vi "ROIsToPoints.vi"(9 "GridPoints":dbl=5.0, 10 "Scan Settings":T2, 11 "ROI":T1(array[cluster])) -> (0 "X-Y Motion Points":i32[][](array[numeric]), 1 "Number of motion points":i32, 2 "Number of points":i32, 3 "Points":i32[][](array[numeric]), 4 "Y-Z Motion Points":i32[][](array[numeric]))   [LabVIEW 2014]
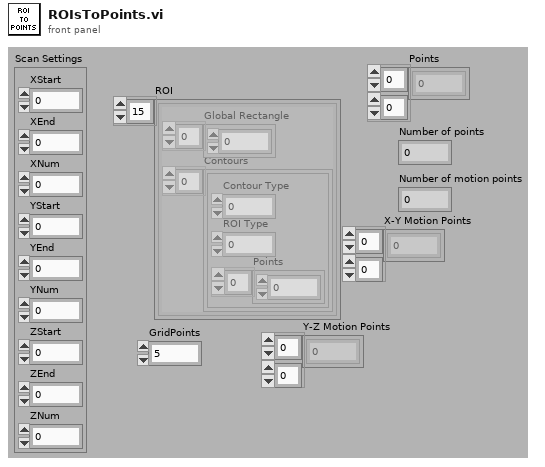
[diagram p1: front panel]
types:
  T1 = cluster{"Global Rectangle":i32[], "Contours":cluster{"Contour Type":u32, "ROI Type":u32, "Points":i32[]}[]}[]
  T2 = cluster{"XStart":i32, "XEnd":i32, "XNum":i32, "YStart":i32, "YEnd":i32, "YNum":i32, "ZStart":i32, "ZEnd":i32, "ZNum":i32}
  T3 = cluster{"Contour Type":u32, "ROI Type":u32, "Points":i32[]}[]
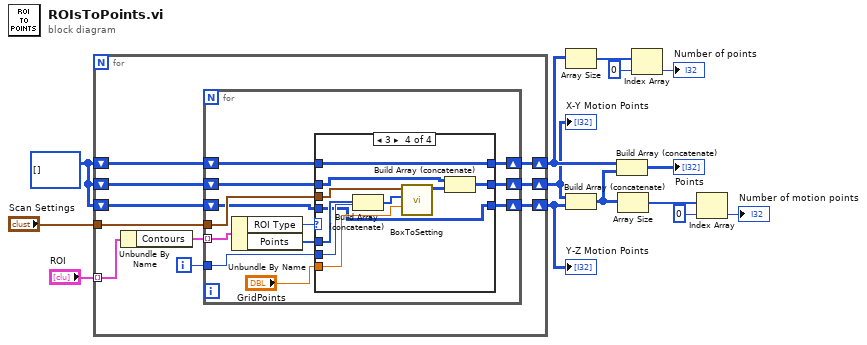
[diagram p0: block diagram]
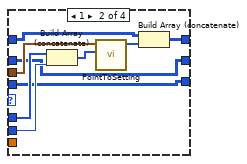
[diagram p3: hidden frame]
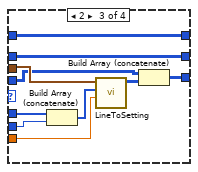
[diagram p4: hidden frame]
diagram:
  w4 = i32[][] []
  n1 = for {
    tunnel: "ROI" -> [w24] mode=indexing
    shift-right: [w20] -> w9
    shift-left: w4 -> [w21]
    tunnel: "Scan Settings" -> [w19]
    shift-right: [w15] -> w3
    shift-left: w4 -> [w18]
    shift-right: [w16] -> w2
    shift-left: w4 -> [w17]
    i -> [w22]
    n2 = Unbundle By Name(w24) -> ("Contours"=w23:T3)
    n3 = for {
      tunnel: w23 -> [w36] mode=indexing
      tunnel: w22 -> [w32]
      shift-right: [w31] -> w20
      shift-left: w21 -> [w33]
      tunnel: w19 -> [w30]
      shift-right: [w25] -> w15
      shift-left: w18 -> [w26]
      shift-right: [w27] -> w16
      shift-left: w17 -> [w28]
      n4 = Unbundle By Name(w36) -> ("ROI Type"=w35:u32, "Points"=w34:i32[])
      n5 = case shown="3" w35 {
        tunnel: w34 -> [_ w48 w58 w67]
        tunnel: w33 -> [w39 w46 w50 w59]
        tunnel: w32 -> [_ w47 w57 w68]
        tunnel: [w39 w45 w50 w59] -> w31
        tunnel: w30 -> [_ w43 w56 w66]
        tunnel: "GridPoints" -> [_ _ w54 w64]
        tunnel: w28 -> [w38 w41 w52 w62]
        tunnel: [w38 w41 w51 w62] -> w27
        tunnel: w26 -> [w37 w40 w49 w61]
        tunnel: [w37 w40 w49 w60] -> w25
        frame 0, Default {
        }
        frame 1 {
          n6 = Build Array (concatenate)(w48, w47) -> (w42:i32[])
          n7 = call "PointToSetting.vi"("Clicked"=w42, "Scan Settings"=w43) -> ("Setting"=w44:i32[])  [unwired: 9 in]
          n8 = Build Array (concatenate)(w46, w44) -> (w45:i32[][])
        }
        frame 2 {
          n9 = Build Array (concatenate)(w58, w57) -> (w55:i32[])
          n10 = call "LineToSetting.vi"("GridSize"=w54, "Line"=w55, "Scan Settings"=w56) -> ("Settings"=w53:i32[][])  [unwired: 8 in]
          n11 = Build Array (concatenate)(w52, w53) -> (w51:i32[][])
        }
        frame 3 {
          n12 = Build Array (concatenate)(w67, w68) -> (w65:i32[])
          n13 = call "BoxToSetting.vi"("GridSize"=w64, "Line"=w65, "Scan Settings"=w66) -> ("Settings"=w63:i32[][])  [unwired: 8 in]
          n14 = Build Array (concatenate)(w61, w63) -> (w60:i32[][])
        }
      }
    }
  }
  "X-Y Motion Points" <- w3
  "Y-Z Motion Points" <- w2
  n15 = Array Size(array=w9) -> (size(s)=w12:i32[])
  n16 = Build Array (concatenate)(w3, w2) -> (w1:i32[][])
  n17 = Build Array (concatenate)(w9, w1) -> (→"Points":i32[][])
  n18 = Array Size(array=w1) -> (size(s)=w7:i32[])
  n19 = Index Array(array=w12, index=0) -> (element=→"Number of points":i32)
  n20 = Index Array(array=w7, index=0) -> (element=→"Number of motion points":i32)
